vi "ryTimerEx Custom Callback.vi"(10 "Message":string, 11 "Destination Refnum":string) -> ()   [LabVIEW 2021]
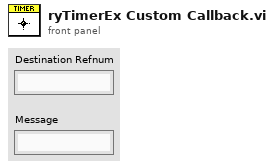
[diagram p1: front panel]
types:
  T1 = cluster{"Message":enum16{"INIT", "EXIT"}, "Data":variant}
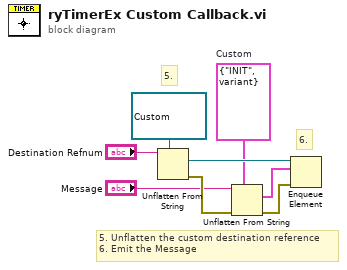
[diagram p0: block diagram]
diagram:
  w2 = T1 {"Message"=enum."INIT", "Data"=variant}  # Custom
  # "6."
  # "5."
  # "5. Unflatten the custom destination reference\n6. Emit the Message"
  n1 = Unflatten From String(type=refnum<queue> refnum ("queue out"), binary string="Destination Refnum") -> (value=w7:refnum<queue>, error out=w6:errorcluster)  [unwired: 3 in, 1 out]
  n2 = Unflatten From String(type=w2, binary string="Message", error in (no error)=w6) -> (value=w1:T1, error out=w4:errorcluster)  [unwired: 2 in, 1 out]
  n3 = Enqueue Element(queue=w7, element=w1, error in (no error)=w4) -> ()  [unwired: 1 in, 3 out]
